vi "Set Image Flip.vi"(10 "iVFlip":i32, 11 "iHFlip":i32) -> (3 "function return":u32)   [LabVIEW 2018, in "AndorSDK.lvlib"]
doc: "EXPNETTYPE unsigned int WINAPI SetImageFlip(int iHFlip, int iVFlip);"
uses:
  AndorSDK.lvlib
  ATMCD32D.dll
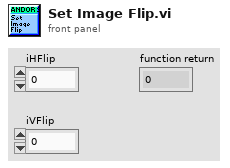
[diagram p1: front panel]
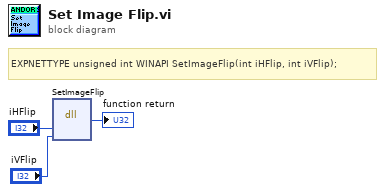
[diagram p0: block diagram]
diagram:
  # "EXPNETTYPE unsigned int WINAPI SetImageFlip(int iHFlip, int iVFlip);"
  n1 = dll-call lib="PTH2babs E\nPersönliches02 - Arbeit03-HiwijobsLabviewCodelibANDOR\tAndor SDK\nATMCD32D.*" fn="SetImageFlip"("iHFlip"="iHFlip", "iVFlip"="iVFlip") -> (→"function return":u32)  [unwired: 5 in, 2 out]
